vi "Read Menu Items.vi"(8 "error in (no error)":errorcluster, 11 "Front Panel Menu in":refnum<class "Front Panel Menu.lvclass">) -> (0 "error out":errorcluster, 2 "Menu Items":T1, 3 "Front Panel Menu out":refnum<class "Front Panel Menu.lvclass">)   [LabVIEW 2024, in "Front Panel Menu.lvclass"]
uses:
  Front Panel Menu.lvclass
  Type Def/Menu Item Group.ctl
  Type Def/Menu Item.ctl
  Front Panel Menu.lvclass/Front Panel Menu.ctl
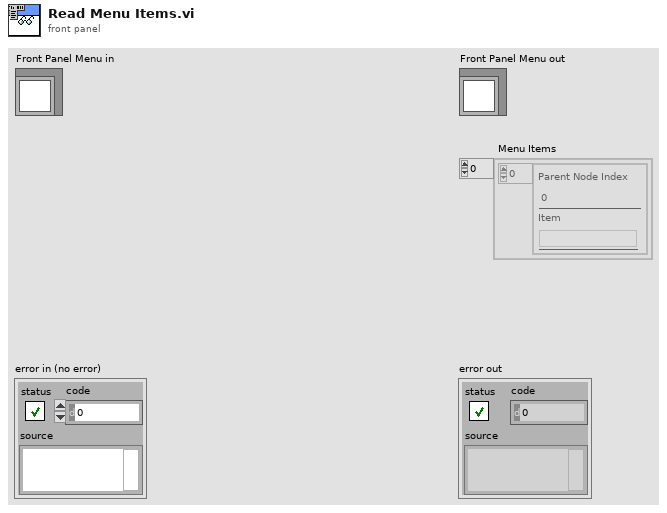
[diagram p1: front panel]
types:
  T1 = typedef "Menu Item Group.ctl" = cluster{"Array":T2[]}[]
  T2 = typedef "Menu Item.ctl" = cluster{"Parent Node Index":i32, "Item":string}
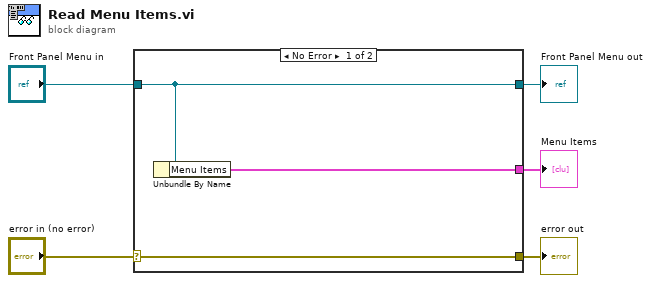
[diagram p0: block diagram]
diagram:
  n1 = case shown="No Error" "error in (no error)" {
    selector: "error in (no error)" -> [w8 w9]
    tunnel: [w8 w9] -> w4
    tunnel: [w7 w10] -> w2
    tunnel: "Front Panel Menu in" -> [w7 w10]
    tunnel: [w6 _] -> w1
    frame No Error {
      n2 = Unbundle By Name(w7) -> ("Menu Items"=w6:T1)
    }
    frame Error {
    }
  }
  "error out" <- w4
  "Front Panel Menu out" <- w2
  "Menu Items" <- w1
